vi "JK Latch.vi"(5 "Reset":bool, 7 "Set":bool) -> (2 "Q":bool)   [LabVIEW 2015]
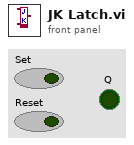
[diagram p1: front panel]
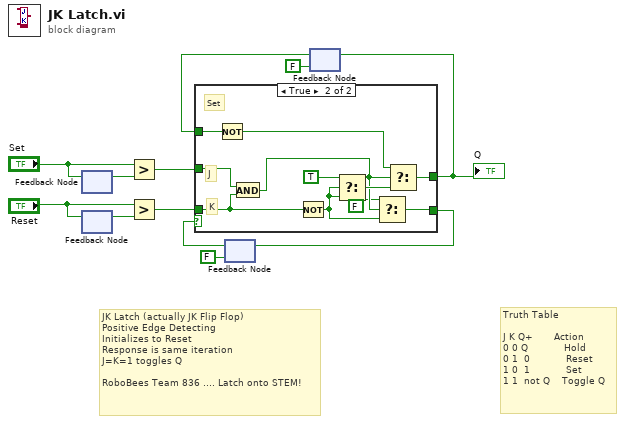
[diagram p0: block diagram]
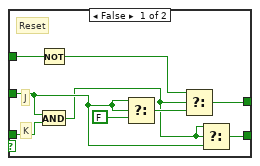
[diagram p2: hidden frame]
diagram:
  # "Truth Table\n\nJ K Q+       Action\n0 0 Q            Hold\n0 1  0            Reset\n1 0  1            Set\n1 1  not Q    Toggle Q"
  # "JK Latch (actually JK Flip Flop)\nPositive Edge Detecting\nInitializes to Reset\nResponse is same iteration\nJ=K=1 toggles Q\n\nRoboBees Team 836 .... Latch onto STEM!"
  n1 = feedback-in #1("Set") -> ()
  n2 = feedback #1() -> (w5:bool)  [unwired: 1 in]
  n3 = feedback #2() -> (w3:bool)  [unwired: 1 in]
  n4 = feedback-in #2("Reset") -> ()
  n5 = Greater?(x="Set", y=w5) -> (0:w4:bool)
  n6 = Greater?(x="Reset", y=w3) -> (0:w2:bool)
  n7 = feedback #3(FALSE) -> (w11:bool)
  n8 = feedback #4(FALSE ("Reset")) -> (w8:bool)
  n9 = case shown="True" w11 {
    tunnel: [w14 w25] -> w10
    tunnel: w2 -> [w20 w30]
    tunnel: w4 -> [w15 w31]
    tunnel: [w18 w29] -> w9
    tunnel: w8 -> [w17 w28]
    frame False {
      # "K"
      # "J"
      # "Reset"
      n10 = Not(x=w17) -> (.not. x?=w16:bool)
      n11 = And(x=w15, y=w20) -> (x .and. y?=w13:bool)
      n12 = Select(t=w15, s=w15, f=FALSE ("Reset")) -> (s? t:f=w19:bool)
      n13 = Select(t=w16, s=w13, f=w19) -> (s? t:f=w18:bool)
      n14 = Select(t=w13, s=w13, f=w15) -> (s? t:f=w14:bool)
    }
    frame True {
      # "K"
      # "J"
      # "Set"
      n15 = Not(x=w28) -> (.not. x?=w27:bool)
      n16 = And(x=w31, y=w30) -> (x .and. y?=w24:bool)
      n17 = Not(x=w30) -> (.not. x?=w22:bool)
      n18 = Select(t=TRUE ("Reset"), s=w22, f=w22) -> (s? t:f=w26:bool)
      n19 = Select(t=FALSE ("Reset"), s=w24, f=w22) -> (s? t:f=w25:bool)
      n20 = Select(t=w27, s=w24, f=w26) -> (s? t:f=w29:bool)
    }
  }
  "Q" <- w9
  n21 = feedback-in #3(w10) -> ()
  n22 = feedback-in #4(w9) -> ()
